vi "Write Current Execution Count.vi"(8 "error in (no error)":errorcluster, 10 "Current Execution Count":u32, 11 "Completion Notification Msg in":refnum<class "Completion Notification Msg.lvclass">) -> (0 "error out":errorcluster, 3 "Completion Notification Msg out":refnum<class "Completion Notification Msg.lvclass">)   [LabVIEW 2023, in "Async Methods Actor.lvlib" / "Completion Notification Msg.lvclass"]
uses:
  Completion Notification Msg.lvclass
  Completion Notification Msg.lvclass/Completion Notification Msg.ctl
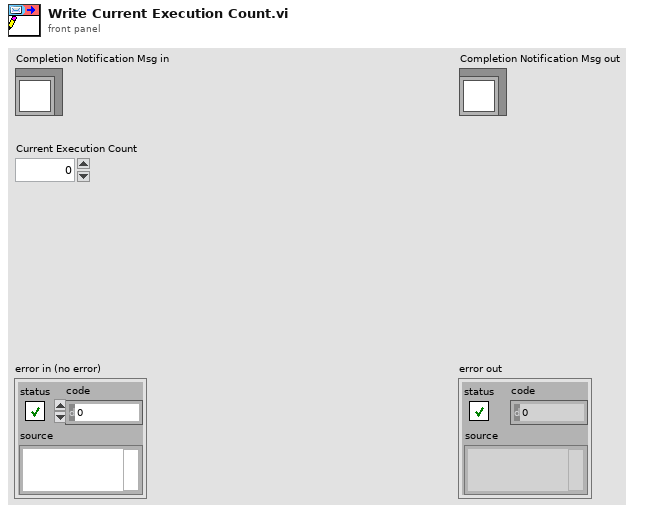
[diagram p1: front panel]
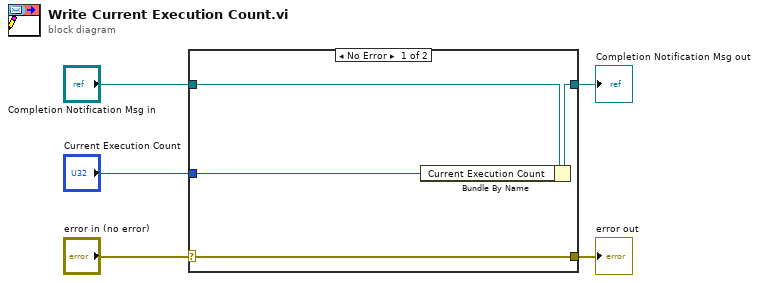
[diagram p0: block diagram]
diagram:
  n1 = case shown="No Error" "error in (no error)" {
    selector: "error in (no error)" -> [w9 w10]
    tunnel: [w9 w10] -> w4
    tunnel: [w7 w11] -> w2
    tunnel: "Completion Notification Msg in" -> [w8 w11]
    tunnel: "Current Execution Count" -> [w6 _]
    frame No Error {
      n2 = Bundle By Name(cluster=w8, "Current Execution Count"=w6) -> (w7:refnum<class "Completion Notification Msg.lvclass">)
    }
    frame Error {
    }
  }
  "error out" <- w4
  "Completion Notification Msg out" <- w2
